vi "BareBone_AcquisitionInterface.vi"() -> ()   [LabVIEW 2011]
panel:
  out "File size (MB)":dbl=160.15164184570312 format="%#.1f"
  out "size":i32=41982792
  in  "Acquire":bool
  out "Timestamps":u32[](array[numeric]) format="%x"
  out "FPGA TS":errorcluster
  in  "Save timestamp data to:":path=path "C:/Data/Antonio/data/manta/2016-12-01/low-light_N2Top_N5Bott_FPGA96ch.dat"
  # "Acquire"
  # "Stop"
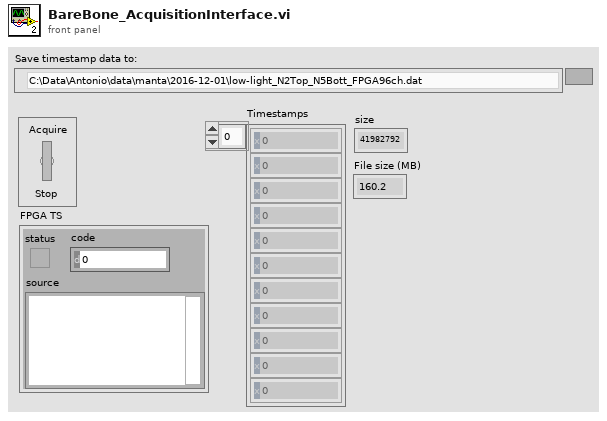
[diagram p1: front panel]
types:
  T1 = typedef "FPGA_reference.ctl" = refnum<k20>
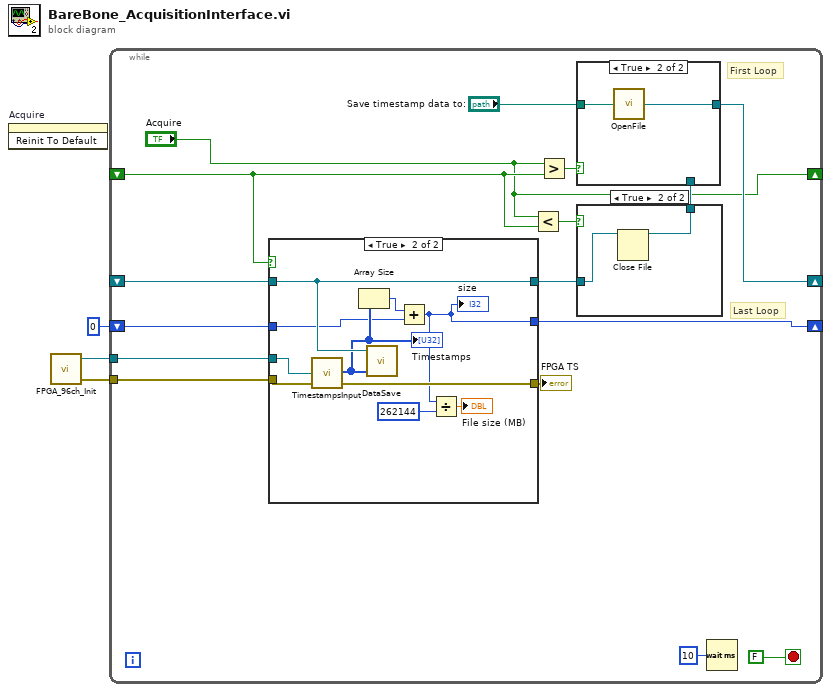
[diagram p0: block diagram]
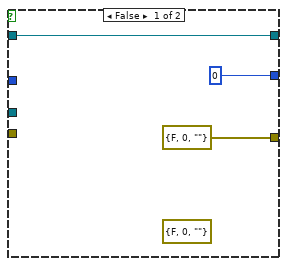
[diagram p4: hidden frame]
diagram:
  n1 = invoke on="Acquire" class="Bool (strict)" method="Reinit To Default"() -> ()  [unwired: 3 in, 3 out]
  n2 = call "FPGA_96ch_Init.vi"() -> ("error out"=w3:errorcluster, "FPGA VI Reference OUt"=w2:T1)  [unwired: 4 in]
  n3 = while {
    shift-right: [w12] -> _
    shift-left: _ -> [w19]
    shift-right: ["Acquire"] -> _
    shift-left: _ -> [w18]
    tunnel: w3 -> [w7]
    tunnel: w2 -> [w6]
    shift-right: [w4] -> _
    shift-left: 0 -> [w5]
    stop <- FALSE stop-if-true
    # "Last Loop"
    # "First Loop"
    n4 = case shown="True" w18 {
      tunnel: w19 -> [w27 w37]
      tunnel: [w27 w37] -> w16
      tunnel: [errorcluster {"status"=FALSE, "code"=0, "source"=""} ("error out") w36] -> w9
      tunnel: w7 -> [_ w35]
      tunnel: w6 -> [_ w34]
      tunnel: w5 -> [_ w31]
      tunnel: [0 w30] -> w4
      frame False {
        (unwired) errorcluster {"status"=FALSE, "code"=0, "source"=""} ("error out")
      }
      frame True {
        n5 = call "TimestampsInput.vi"("error in"=w35, "FPGA VI Reference In"=w34) -> ("error out"=w36:errorcluster, "Data"=w33:u32[])  [unwired: 2 in]
        "Timestamps" <- w33
        n6 = Array Size(array=w33) -> (size(s)=w32:i32)
        n7 = call "DataSave.vi"("Data"=w33, "File Refnum"=w37) -> ()  [unwired: 4 in]
        n8 = Add(x=w32, y=w31) -> (x+y=w30:i32)
        "size" <- w30
        n9 = Divide(x=w30, y=262144) -> (x/y=→"File size (MB)":dbl)
      }
    }
    "FPGA TS" <- w9
    n10 = Less?(x="Acquire", y=w18) -> (x < y?=w17:bool)
    n11 = Greater?(x="Acquire", y=w18) -> (0:w14:bool)
    n12 = case shown="True" w17 {
      tunnel: w16 -> [w23 w24]
      tunnel: [w23 w24] -> w11
      frame False {
      }
      frame True {
        n13 = Close File(refnum=w24) -> ()  [unwired: 1 in, 2 out]
      }
    }
    n14 = case shown="True" w14 {
      tunnel: "Save timestamp data to:" -> [_ w22]
      tunnel: [w20 w21] -> w12
      tunnel: w11 -> [w20 _]
      frame False {
      }
      frame True {
        n15 = call "OpenFile.vi"("Filename"=w22) -> ("File Refnum"=w21:refnum<file>)  [unwired: 4 in]
      }
    }
    n16 = Wait (ms)(milliseconds to wait=u32 10) -> ()  [unwired: 1 out]
  }
